vi "AlliGator Decay Fit Parameter Map Context Menu Handler.vi"(8 "Error In":errorcluster, 9 "Decay Fit Parameter":T1, 11 "Image Event Data":T2) -> (0 "Error Out":errorcluster, 3 "AlliGator Actions":T5[](array[typedef]))   [LabVIEW 2021, in "AlliGator Decay Fit Parameter Map.lvlib"]
doc: "Decay Fit Parameter Map contextual menu handler."
uses:
  AlliGator Decay Fit Parameter Map.lvlib
  Action Engine/AlliGator Q Element.ctl
  Action Engine/AlliGator Q Event.ctl
  Image/Image Display Event.ctl
  Image/Image Control Refnum.ctl
  <vilib>/Utility/miscctls.llb/LVPoint32TypeDef.ctl
  Image/Image Display to Clipboard Options.ctl
  Fits/IRF(X)PSED/Decay Fit Parameters & Derived Quantities List v2.ctl
  Globals, Variables, Constants/AlliGator Variables List.ctl
  Files/Load-Save File Info.ctl
  Variant/Variant to Data/Variant to I32.vi
  Action Engine/AlliGator Action Engine.lvlib
  Image/Image.lvlib
  Files/Files.lvlib
  Globals, Variables, Constants/AlliGator Globals, Variables & Constants.lvlib
  Variant/Variant to Data/Variant to Data.lvlib
  Fits/Fits.lvlib
  AlliGator Decay Parameter Map Update Event Data.ctl
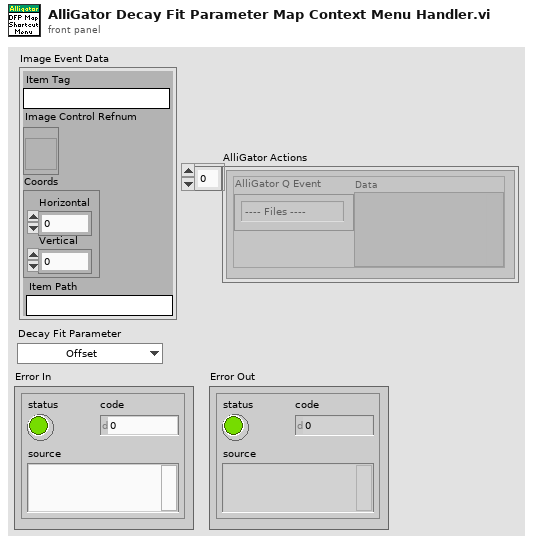
[diagram p1: front panel]
types:
  T1 = typedef "Fits.lvlib/Decay Fit Parameters & Derived Quantities List v2.ctl" = enum16{"Offset", "Baseline", "A_1", "tau_1", "A_2", "tau_2", "<tau>_a", "f1_a", "f2_a", "<tau>_i", "f1_i", "f2_i", "-", "R^2", "Chi^2"}
  T2 = typedef "Image.lvlib/Image Display Event.ctl" = cluster{"Item Tag":string, "Image Control Refnum":T3, "Coords":T4, "Item Path":string}
  T3 = typedef "Image.lvlib/Image Control Refnum.ctl" = refnum<vi>
  T4 = typedef "LVPoint32TypeDef.ctl" = cluster{"Horizontal":i32, "Vertical":i32}
  T5 = typedef "AlliGator Action Engine.lvlib/AlliGator Q Element.ctl" = cluster{"AlliGator Q Event":T6, "Data":variant}
  T6 = typedef "AlliGator Action Engine.lvlib/AlliGator Q Event.ctl" = enum16{"---- Files ----", "Files:Set Batch Export Files To Save", "Files:Set Dataset Loading & Pre-processing Options", "Files:Check #Frames in Dataset", "Files:Increment Frame Index", "Files:Open Mask Image", "Files:Open White Light Image", "Files:Open Single Dataset", "Files:New Folder of Folders Selected", "Files:Load File (all Types)_Scriptable", "Files:Move Flattened Series to Folders Series", "Files:Select Folder", "Files:Load FLI Dataset", "Files:Load Swiss SPAD 1 Dataset", "Files:Load Swiss SPAD 2 Dataset", "Files:Load .sdt FLI Dataset", "Files:Load .ptu FLI Dataset", "Files:Load .bin FLI Dataset", "Files:Load Single Gate Image Folder", "Files:Load I/m/phi Dataset (deprecated)", "Files:Load Single Image", "Files:Subtract Background File", "Files:Export FLI Dataset", "Files:Load HDF5 FLI Dataset", "Files:Set Destination File Path", "Files:Save Mask Image", "Files:Batch Conversion", "Files:New Folder Selected", "Files:Close FLI Dataset", "Files:Close FLI Dataset Series", "Files:Close White Light Image", "Files:Close Mask Image", "---- FLI Dataset ----", "FLI Dataset:Channel Arithmetic", "FLI Dataset:Export Average Lifetime Map as ASCII", "FLI Dataset:Export User-Defined Quantity Map as ASCII", "FLI Dataset:Python Function FLI Dataset Event", "FLI Dataset:ROI Analysis", "FLI Dataset:Tilted Logistic Square Gated IRF Characteristics Map", "FLI Dataset:Logistic Square Gated IRF Characteristics Map", "FLI Dataset:Square Gated IRF Characteristics Map", "FLI Dataset:Multi-ROI Single-Pixel Phasor Analysis", "FLI Dataset:Multi-ROI Single-Pixel NLSF Analysis", "FLI Dataset:All ROIs IRF Extraction", "FLI Dataset:All ROIs Decay Fit Non-Interactive (Fast + Individual IRF)", "FLI Dataset:All ROIs Phasor Analysis", "FLI Dataset:All ROIs Decay Fit", "FLI Dataset:Fluorescence Decay Statistics", "FLI Dataset:Update Decay Statistics Graph", "FLI Dataset:Get Decay from ROI", "FLI Dataset:All ROIs Average Lifetimes", "FLI Dataset:Save/Load Local IRFs", "FLI Dataset:Clear Local IRFs", "---- FLI Dataset Series ----", "FLI Dataset Series:Sum All Datasets in Series", "FLI Dataset Series:Add Dataset to Accumulated Dataset", "FLI Dataset Series:Display Accumulated Dataset", "FLI Dataset Series:Clear Dataset Series Sum", "FLI Dataset Series:Time-Series Analysis (NLSF)", "FLI Dataset Series:Time-Series Analysis (Phasor)", "---- Image ----", "Image:Update Image Profile Plots", "Image:Image Histogram Cursor Move", "Image:Image Histogram", "Image:Image Contrast", "Image:Set Image Histogram Cursor Move Flag", "Image:Clear Image Overlay", "Image:Use ROI as Search Area", "Image:Set ROI Diameter", "Image:Save Image Data as TIFF", "Image:Save Displayed Image with Overlay", "Image:Save Image Overlay Only", "Image:Save Image as Hot Pixel Mask", "Image:Change Source Image Color Palette", "Image:Copy Image to Clipboard", "Image:Source Image ROI Selection", "Image:Delete All ROIs", "Image:Delete All Unselected ROIs", "Image:Delete ROI", "Image:Merge All ROIs", "Image:Store ROI", "Image:Source Image ROI Storage", "Image:Export ROI Description to Notebook", "Image:Save ROI", "Image:Load ROI", "Image:Paste ROI Definition", "Image:Clear ROI", "Image:Identify ROIs in Mask Image", "Image:Create Complementary ROI", "Image:Create Contour ROI", "Image:Create ROI(s) from Pixels with Peak above Min_Scriptable", "Image:Create ROI(s) from Pixels with Intensity above Min_Scriptable", "Image:Compute ROI Statistics", "Image:Delete ROI(s) based on ROI Characteristics", "Image:Create ROI Grid", "Image:ROI to Individual Pixel ROIs", "Image:Python Function Source Image Event", "Image:Show Phasor Calibration Map ROI Centers", "Image:Convert ROI to Mask Image", "Image:Mouse Move", "Image:Mouse Up", "Image:Set Source Image Mouse Move Flag", "Image:Add Scale Bar Overlay", "Image:Delete Existing ROIs Option", "Image:Overlay ROI Median", "Image:Check Current ROI", "---- Decay ----", "Decay:Clear IRF/Reference Plot", "Decay:Add Decay to Graph", "Decay:Smoothen Plot", "Decay:Smoothen Plot Tail", "Decay:Average Selected Plots", "Decay:Extract IRF", "Decay:Optimal IRF Extraction", "Decay:Threshold IRF", "Decay:Fit to Model IRF", "Decay:Fit IRF to Square Gate", "Decay:Fit IRF to Logistic Square Gate", "Decay:Fit IRF to Tilted Logistic Square Gate", "Decay:Create Bounding Cursors Set", "Decay:Export Bounding Cursors Definition to Notebook", "Decay:Denoise Plot", "Decay:Compute Cumulative Function", "Decay:Use as Reference Decay", "Decay:Show Reference Decay/IRF", "Decay:Extrapolate Decay", "Decay:Create Head & Tail Bounding Cursors", "Decay:Store Cursor-defined Head & Tail Fractions", "Decay:Rebin Plot", "Decay:1-Normalize Decay", "Decay:[0-1]-Normalize Plot", "Decay:Straighten Decay", "Decay:Shift Decay", "Decay:Fold Decay", "Decay:Fit Decay", "Decay:Global Fit of Selected Decays", "Decay:Post Global Fit Script", "Decay:Add Global Fit Parameters to Graph", "Decay:Add Decay Parameter(s) to Plot (Graph)", "Decay:Export Decay to Phasor Graph", "Decay:Plot Decay Shifts", "Decay:Compute Average Lifetime", "Decay:Plot Convolution", "Decay:Graph Tip Strip Update", "---- Decay Statistics ----", "Decay Statistics:Tip Strip Update", "---- Intensity Time Trace ----", "Intensity Time Trace:Use File Timestamp", "Intensity Time Trace:Load Intensity Corrections File", "Intensity Time Trace:Clear Intensity Corrections File", "Intensity Time Trace:Tip Strip Update", "---- Phasor Plot ----", "Phasor Plot:Build Phasor Plot", "Phasor Plot:Change Phasor Plot Color Palette", "Phasor Plot:Adjust Phasor Plot Display Range", "Phasor Plot:Highlight Image ROI in Phasor Plot", "Phasor Plot:Save Phasor Plot Image with Overlay", "Phasor Plot:Export Complex Phasor Map", "Phasor Plot:Export Phasor Ratio Map", "Phasor Plot:Export Average Lifetime Map", "Phasor Plot:Compute Phase Lifetime Histogram", "Phasor Plot:Compute Phasor Ratio Histogram", "Phasor Plot:Compute Phase Lifetime vs Intensity Scatter Plot", "Phasor Plot:Weber 2-Component Decomposition", "Phasor Plot:Update Phasor Color Map Vertices", "Phasor Plot:Clear Phasor Overlay", "Phasor Plot:Use Segment Extremities as References", "Phasor Plot:Use UC/Segment Intersections as References", "Phasor Plot:Use UC/Principal Axis Intersections as References", "Phasor Plot:Use UC/Linear Fit Intersections as References", "Phasor Plot:Update Phasor Plot Reference", "Phasor Plot:Show Local Phasor Info in Phasor Plot", "Phasor Plot:Update Phasor Plot State", "Phasor Plot:Phasor Plot ROI Storage", "Phasor Plot:Phasor Plot ROI Selection", "Phasor Plot:Python Function Phasor Plot Event", "Phasor Plot:Overlay Phasor ROI, Ratio or Map in Source Image", "Phasor Plot:Compute Decay of Selected Phasors", "Phasor Plot:Phasor at Image Pixel", "Phasor Plot:Mouse Move", "Phasor Plot:Mouse Up", "Phasor Plot:Display Range Mouse Move", "Phasor Plot:Set Mouse Move Flag", "---- Phasor Graph ----", "Phasor Graph:Calibrated Phasor Map Series", "Phasor Graph:Whole Image Phasor Scatter Plot (deprecated)", "Phasor Graph:Get Phasor Value", "Phasor Graph:Create New Phasor Plot Dialog", "Phasor Graph:Update Last Phasor Value", "Phasor Graph:Update Phasor (m, phi)", "Phasor Graph:Remove Single Phasor from Plot", "Phasor Graph:Add Single Phasor to Plot", "Phasor Graph:Remove Phasor Plot", "Phasor Graph:Remove Selected Phasor Plots", "Phasor Graph:Clear Phasor Data", "Phasor Graph:Clear Phasor Graph", "Phasor Graph:Cursor Move", "Phasor Graph:Draw Cursor Connecting Line", "Phasor Graph:Clear Cursor Connecting Line", "Phasor Graph:Find UC Intersection", "Phasor Graph:Use UC/Cursor-Defined Line Intersections", "Phasor Graph:Use Selected Plots Fitted Line/UC Intersections", "Phasor Graph:Use Selected Plots Principal Axis/UC Intersections", "Phasor Graph:Show Single Phasor", "Phasor Graph:Save Single Phasor Plot", "Phasor Graph:Save All Phasor Plots", "Phasor Graph:Load Phasor Plot(s)", "Phasor Graph:Phasor Multiplication", "Phasor Graph:Compute Average Phasor", "Phasor Graph:Compute Multiple Average Phasors (Selected Plots)", "Phasor Graph:Export Single Phasor Plot Phase Lifetimes", "Phasor Graph:Phase Lifetime Trajectory (deprecated)", "Phasor Graph:Phase Lifetime vs Intensity Scatter Plot (deprecated)", "Phasor Graph:Parameter 2 vs Parameter 1 Scatter Plot", "Phasor Graph:Use Cursor n Location", "Phasor Graph:Set Reference n to Current Phase Lifetime Value", "Phasor Graph:Set Reference n to Lifetime Value", "Phasor Graph:Set Cursor n Location", "Phasor Graph:Save Phasor Graph Image", "Phasor Graph:Update SEPL Plot", "Phasor Graph:Export Single Phasor Plot Data", "Phasor Graph:Export Selected Phasor Plots Data", "Phasor Graph:Python Function Phasor Graph Event", "Phasor Graph:Tip Strip Update", "---- Calibration ----", "Calibration:Set Calibration Type", "Calibration:Load/Save Phasor Calibration", "Calibration:Load/Save Phasor Calibration Series", "Calibration:Load/Save Phasor Calibration Map", "Calibration:Use as Calibration", "Calibration:Compute Optimal Calibration from Phasor References", "Calibration:Clear Phasor Calibration", "Calibration:Single Phasor Calibration Information", "Calibration:Use as Calibration Series", "Calibration:Use as Calibration Map", "Calibration:Clear Calibration Series", "Calibration:Phasor Calibration Series Information", "Calibration:Clear Calibration Map", "Calibration:Phasor Calibration Map Information", "Calibration:Apply Phasor Calibration", "Calibration:Update Single Plot Calibration", "Calibration:Update Multiple Plots Calibration", "Calibration:Clear Single Plot Calibration", "Calibration:Clear All Plots Calibrations", "Calibration:Clear Plot(s) Calibration(s)?", "Calibration:Phasor Calibration Maps (# Gates Series)", "---- Phasor Ratio ----", "Phasor Ratio:Clear Reference n", "Phasor Ratio:Toggle Selected Plot(s)  Lock to Reference 1", "Phasor Ratio:Use as Reference n", "Phasor Ratio:Send Reference n to Notebook", "Phasor Ratio:Toggle Selected Plot(s)  Lock to Reference 2", "Phasor Ratio:Compute Phasor Ratio at Mouse Location", "Phasor Ratio:Compute Phasor Plot's Average Phasor Ratio", "Phasor Ratio:Compute Time-Series Phasor Ratios", "Phasor Ratio:Fit Line to Phasor Ratio Plot", "Phasor Ratio:Save References", "Phasor Ratio:Load References", "Phasor Ratio:Update Phasor Reference 1", "Phasor Ratio:Update Phasor Reference 2", "Phasor Ratio:Move Cursor n to Reference n", "Phasor Ratio:Use as Phasor Reference 1 Lifetime", "Phasor Ratio:Use as Phasor Reference 2 Lifetime", "Phasor Ratio:Export Phasor Ratio Map as ASCII", "Phasor Ratio:Tip Strip Update", "---- Lifetime & Other Parameters Graph ----", "Lifetime:Power Law from Intensity Distribution", "---- Decay Fit Parameter Map ----", "Decay Fit Parameter Map:Export ROI NLSF Data as ASCII", "Decay Fit Parameter Map:Set Decay Fit Parameter Map Selection", "Decay Fit Parameter Map:Build Decay Fit Parameter Map", "Decay Fit Parameter Map:Change Decay Fit Parameter Map Color Palette", "Decay Fit Parameter Map:Export Decay Fit Parameter Map Data as ASCII", "Decay Fit Parameter Map:Export All Decay Fit Parameter Maps Data as ASCII", "Decay Fit Parameter Map:Selected Parameter Scatterplot", "Decay Fit Parameter Map:Parameter 2 vs Parameter 1 Scatterplot", "Decay Fit Parameter Map:Save Decay Fit Parameter Map Image", "Decay Fit Parameter Map:Save-Load IRFs & Fit Data", "Decay Fit Parameter Map:Update Local Decay Plots", "Decay Fit Parameter Map:Python Function Decay Fit Parameters Map Event", "Decay Fit Parameter Map:Overlay Decay Fit Parameter Map in Source Image", "Decay Fit Parameter Map:Selected Parameter vs Intensity Scatterplot", "Decay Fit Parameter Map:Mouse Up", "Decay Fit Parameter Map:Display Range Mouse Move", "Decay Fit Parameter Map:Change Map Resolution", "---- Parameter Map ----", "Parameter Map:Export ROI Parameters Data as ASCII", "Parameter Map:Delete Parameter Map Set", "Parameter Map:Update Parameter List", "Parameter Map:Build Parameter Map", "Parameter Map:Change Parameter Map Color Palette", "Parameter Map:Export Parameter Map Data as ASCII", "Parameter Map:Export All Parameter Maps Data as ASCII", "Parameter Map:Selected Parameter Scatterplot", "Parameter Map:Parameter 2 vs Parameter 1 Scatterplot", "Parameter Map:Selected Parameter vs Intensity Scatterplot", "Parameter Map:Save Parameter Map Image", "Parameter Map:Save-Load IRFs & Parameter Maps (TODO)", "Parameter Map:Set Parameter Map Selection", "Parameter Map:Python Function Parameter Map Event", "Parameter Map:Overlay Parameter Map in Source Image", "Parameter Map:Update Local Decay Plots", "Parameter Map:Mouse Up", "Parameter Map:Display Range Mouse Move", "---- Generic Graph ----", "Generic Graph:Generic XY Graph Event", "Generic Graph:Python Function XY Graph Event", "Generic Graph:New Plot", "Generic Graph:Save Plot", "Generic Graph:XY Plot Histogram", "Generic Graph:Set XY Graph Plot Name", "Generic Graph:Set Last Cursor Style", "Generic Graph:Tip Strip Update", "---- GUI ----", "GUI:Start Script", "GUI:Type of Displayed Image Changed", "GUI:Gate Image Slide Changed", "GUI:Show Busy Icon", "GUI:Show Busy Icon & Abort Button", "GUI:Hide Busy Icon", "GUI:Hide Busy Icon & Abort Button", "GUI:Abort", "GUI:End Script", "GUI:Start Timing", "GUI:End Timing", "GUI:Set State Indicator", "GUI:Send Parameters JSON Strings to Clipboard", "GUI:Set Gate Step", "GUI:Idle", "GUI:Initialization", "GUI:Quit", "GUI:Increment Dataset Index", "GUI:Set Dataset Index to -1", "GUI:Time Series Slider Moved", "GUI:Time Series Slider Changed", "GUI:Toggle Playback or Loop", "GUI:Playback Script", "GUI:Set Phasor Frequency", "GUI:Open Window", "GUI:Start Test Script", "GUI:End Test Script", "DEBUG"}
  T7 = typedef "Image.lvlib/Image Display to Clipboard Options.ctl" = cluster{"Include Overlay (T)":bool, "Image Only (T)":bool}
  T8 = cluster{"Fit Parameter 1":T1, "Fit Parameter 2":T1}
  T9 = typedef "AlliGator Globals, Variables & Constants.lvlib/AlliGator Variables List.ctl" = enum16{"---- GUI ----", "GUI:Initialization Status", "GUI:State Indicators Refnum", "GUI:Original AlliGator Menu Items", "GUI:Current Action Loop State", "GUI:Script in progress", "GUI:Playback", "GUI:Loop Playback", "GUI:Search ROI Used", "GUI:Search ROI", "Decay Graph Max Legend Size", "Intensity Graph Max Legend Size", "Decay Statistics Graph Max Legend Size", "Phasor Graph Max Legend Size", "Phasor Ratio Graph Max Legend Size", "Lifetime Graph Max Legend Size", "---- Files ----", "Files:Export Dataset Frames as Individual Files", "Files:Show Batch Export Help Balloons", "Files:Frames in Dataset", "Files:ptu File Frame Start Indices", "Files:Current Frame in Dataset", "Files:Current Frame Timestamp", "Files:Dataset Loaded", "Files:Dataset Metadata", "Files:Dataset Channel", "Files:Dataset Data Description", "Files:Background Dataset Metadata", "Files:Background Dataset Channel", "Files:Background Dataset Data Description", "Files:Background File Subtraction", "Files:Background File Path", "Files:Background File Pile-up Correction", "Files:Background File Pixel Well Capacity", "Files:Background File Scaling Factor", "Files:Current Dataset Load Settings", "Files:Dataset Path", "Files:ICCD-specific Information", "Files:Macrotime Gate Separation", "------ Python Plugins ------", "Python Plugins:Information", "Python Plugins:Python Session", "Python Plugins:Valid Python Session?", "---- Source Image ----", "Source Image:ROIs", "Source Image:Current ROI", "Source Image:ROI Event Refnum", "X_Source Image:Display Range", "X_Source Image:Palette Information", "X_Source Image:Type of Displayed Image", "X_Time Gate Slider", "Source Image:Palette List", "Source Image:Scale", "Source Image:ROI Overlay Color", "Source Image:Overlay to Erase", "Source Image:Is Displayed Image Accumulated", "Source Image:White Light Image Modified", "Source Image:Mask Image Modified", "---- Image Profile Window ----", "Image Profile:Window Event Refnum", "Image Profile:IntensityType", "Image Profile:Intensity Average Type", "Image Profile:Intensity-weighted SDV", "Image Profile:Box Profile Type", "Image Profile:Window Open", "Image Profile:Plotted Fit Parameter", "------ Phasor Graph -------", "Phasor Graph:Show Line", "---- Phasor Plot ---", "Phasor Plot:Parameters Changed", "Phasor Plot:FLI Dataset Modified since last Calculation", "Phasor Harmonics Data", "Selected Phasor Harmonics", "Phasor Harmonic Manager Event Refnum", "Phasor Plot:ROIs", "Phasor Plot:Current ROI", "Phasor Plot:ROI Event Refnum", "Phasor Plot:Image Reference Points", "Phasor Plot:Computed", "Phasor Plot:Palette Information", "Phasor Plot:Palette List", "Phasor Plot:Phasor Ratio Palette Information", "Phasor Plot:Phasor Ratio Palette List", "Phasor Plot:Image Scale", "Phasor Plot:Image Overlay to Erase", "Phasor Plot:Image Elements to Update", "Phasor Plot:Current Calculation Parameters", "Phasor Plot:Current Calibration Options", "Phasor Plot:Reset Cumulated Phasor Plot", "Phasor Plot:Reference 1", "Phasor Plot:Lifetime Reference 1", "Phasor Plot:Reference 1 Frequency", "Phasor Plot:Reference 2", "Phasor Plot:Lifetime Reference 2", "Phasor Plot:Reference 2 Frequency", "---- Decay Analysis ----", "Number of Selected Decays to Fit", "LS Fit Results", "LAR Fit Results", "BS Fit Results", "Last Decay Max - Min", "Best Fit Parameters", "Best Fit Parameter Names", "Actual Size X", "Actual Size Y", "Binning X", "Binning Y", "Actual # Gates", "Dataset Number", "Gates to...", "Gates Skipped", "Gates to keep", "Gate Step", "Gate Separation", "Reversed Gates", "Pile-up Correction", "Pixel Well Capacity", "Background Subtracted", "Background Subtraction Method", "Background Definition Range", "Background File (deprecated)", "Number of Dataset Accumulated", "Array of Accumulated Dataset Paths", "Do Averaged Datasets", "Destination File Path", "Process Plot Target", "Use 1/D as Phasor Frequency", "---- Decay Fit Parameter Map -----", "Decay Fit Parameter Map:Palette Information", "Decay Fit Parameter Map:Palette List", "Decay Fit Parameter Map:X Resolution", "Decay Fit Parameter Map:Y Resolution", "---- Parameter Map ----", "Parameter Map:Palette Information", "Parameter Map:Palette List", "------- Local Decay Window ---------", "Local Decay Graph Window:Event Refnum", "Local Decay Graph Window:Use normalized IRF for convolution", "----- Miscellaneous ----", "Misc:Skippable Dialog Windows Status"}
  T10 = typedef "Files.lvlib/Load-Save File Info.ctl" = cluster{"Load/Save":bool, "File Path":path}
  T11 = typedef "AlliGator Decay Fit Parameter Map.lvlib/AlliGator Decay Parameter Map Update Event Data.ctl" = cluster{"Parameter":T1, "Parameter changed":bool}
  T12 = cluster{"Image Control Refnum":T3, "Image to Clipboard Options":T7}
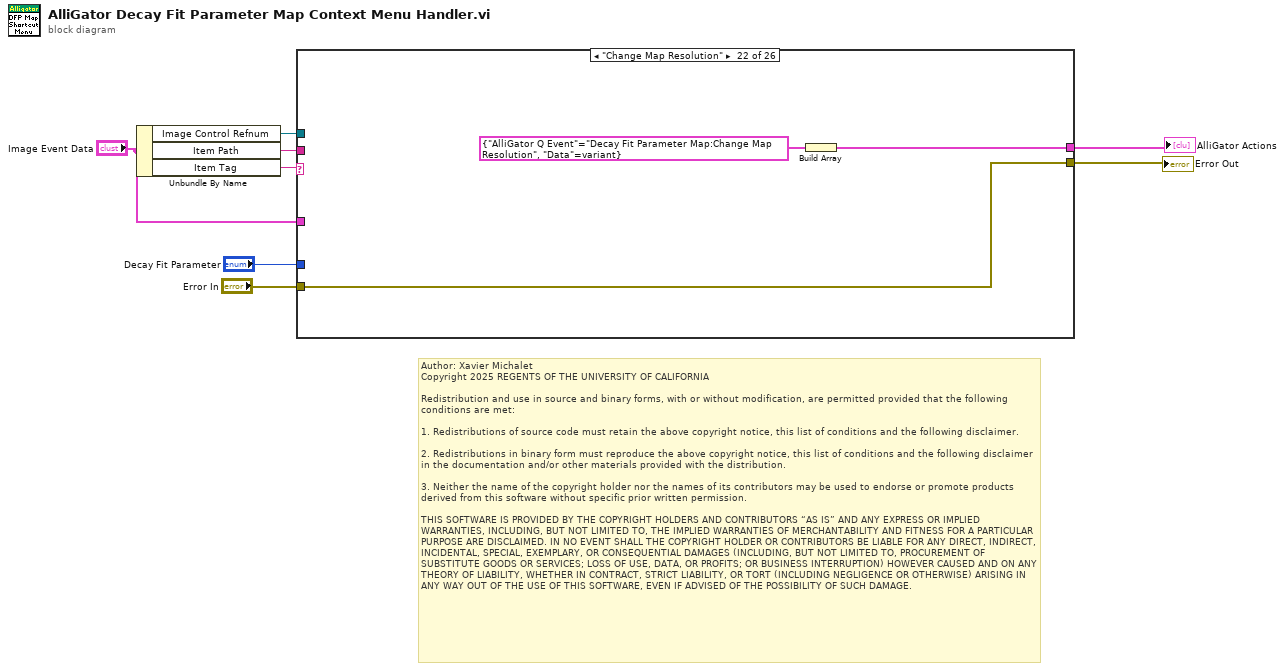
[diagram p0: block diagram]
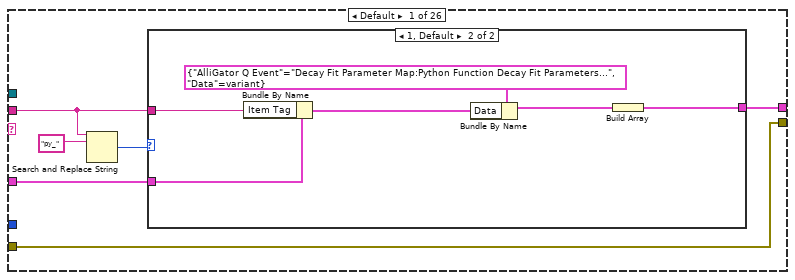
[diagram p2: hidden frame]
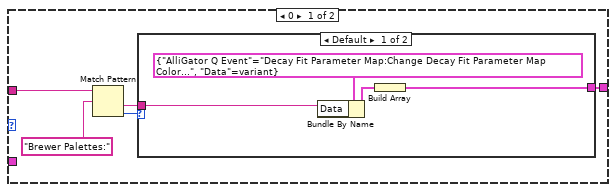
[diagram p3: hidden frame]
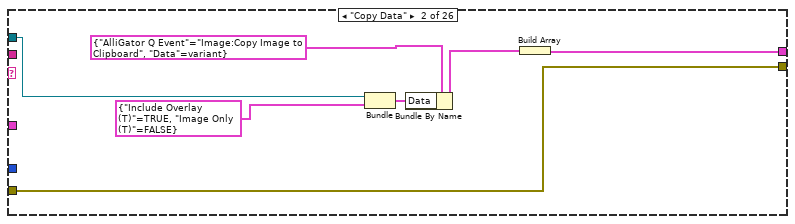
[diagram p5: hidden frame]
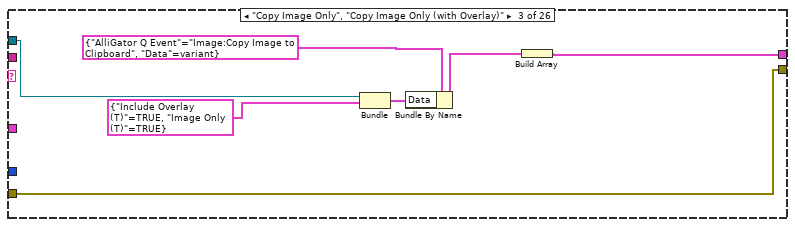
[diagram p6: hidden frame]
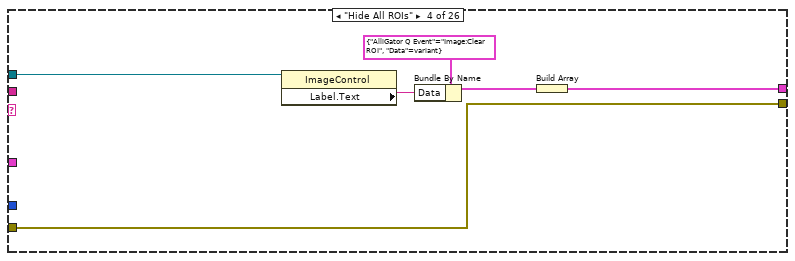
[diagram p7: hidden frame]
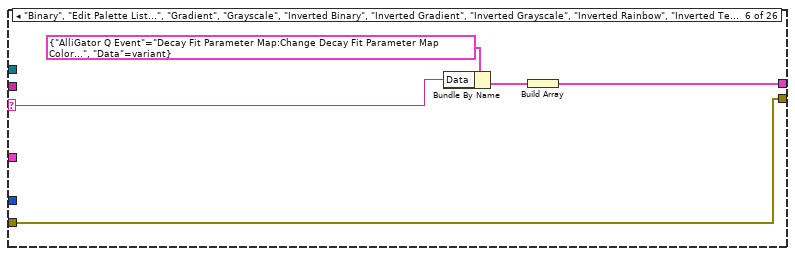
[diagram p9: hidden frame]
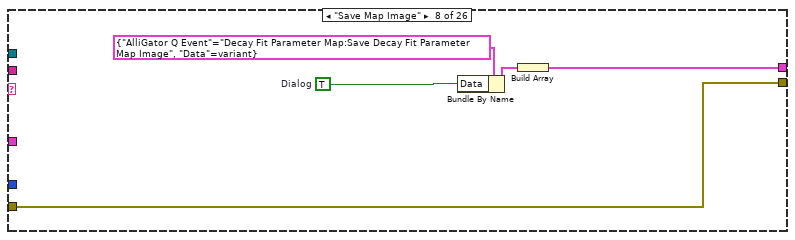
[diagram p11: hidden frame]
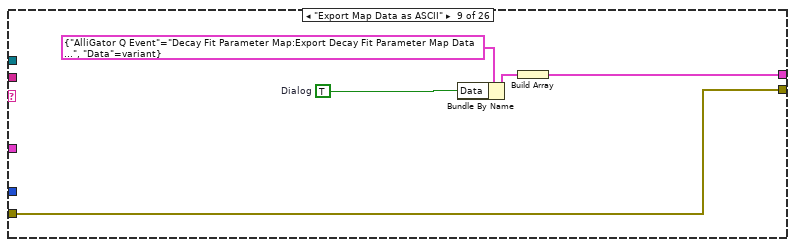
[diagram p12: hidden frame]
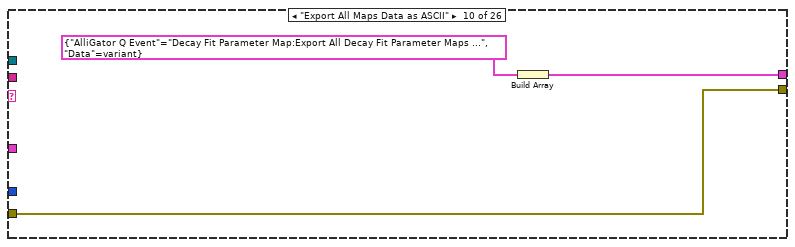
[diagram p13: hidden frame]
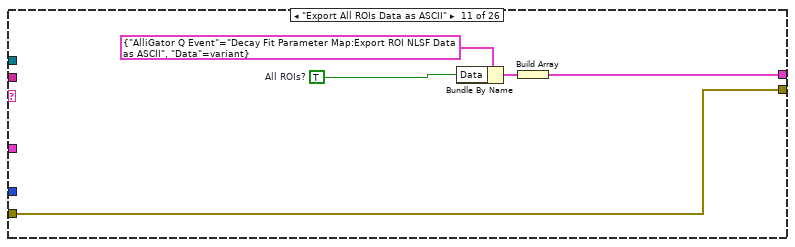
[diagram p14: hidden frame]
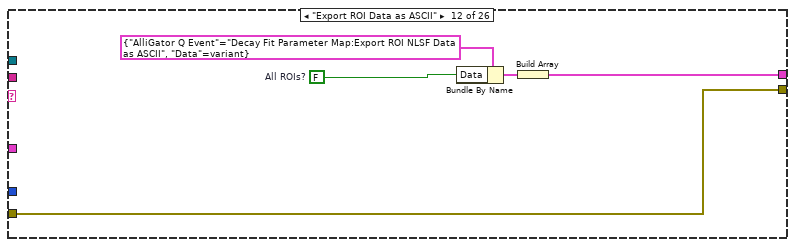
[diagram p15: hidden frame]
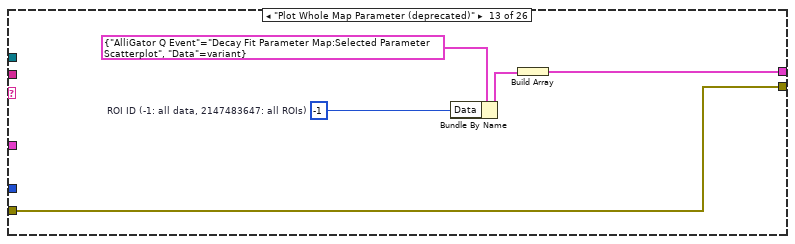
[diagram p16: hidden frame]
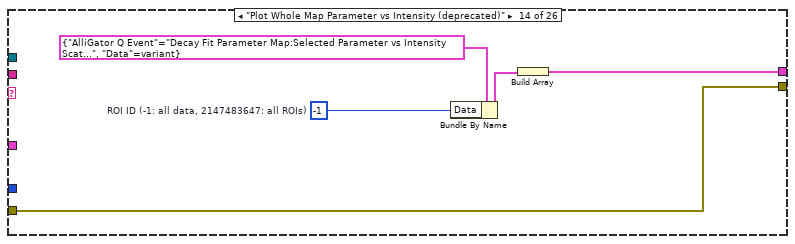
[diagram p17: hidden frame]
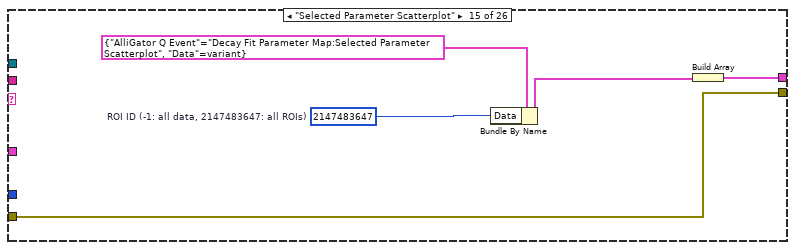
[diagram p18: hidden frame]
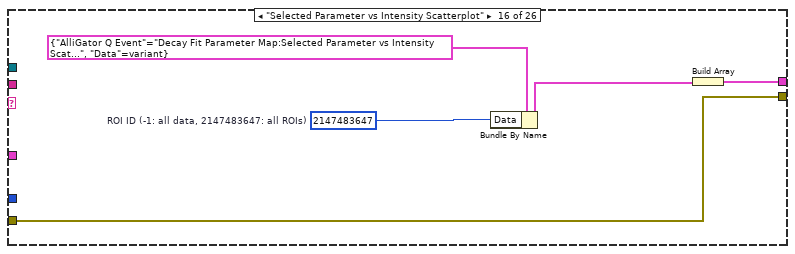
[diagram p19: hidden frame]
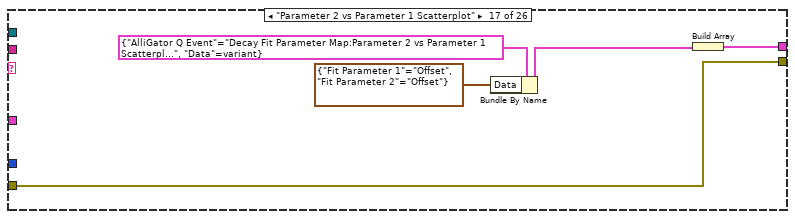
[diagram p20: hidden frame]
diagram:
  # "Author: Xavier Michalet\nCopyright 2025 REGENTS OF THE UNIVERSITY OF CALIFORNIA\n\nRedistribution and use in source and binary forms, with or without modification, are permitted provided that the following conditions are met:\n\n1. Redistributions of source code must retain the above copyright notice, this list of conditions and the following disclaimer.\n\n2. Redistributions in binary form must reproduce the above copyright notice, this list of conditions and the following disclaimer in the documentation and/or other materials provided with the distribution.\n\n3. Neither the name of the copyright holder nor the names of its contributors may be used to endorse or promote products derived from this software without specific prior written permission.\n\nTHIS SOFTWARE IS PROVIDED BY THE COPYRIGHT HOLDERS AND CONTRIBUTORS “AS IS” AND ANY EXPRESS OR IMPLIED WARRANTIES, INCLUDING, BUT NOT LIMITED TO, THE IMPLIED WARRANTIES OF MERCHANTABILITY AND FITNESS FOR A PARTICULAR PURPOSE ARE DISCLAIMED. IN NO EVENT SHALL THE COPYRIGHT HOLDER OR CONTRIBUTORS BE LIABLE FOR ANY DIRECT, INDIRECT, INCIDENTAL, SPECIAL, EXEMPLARY, OR CONSEQUENTIAL DAMAGES (INCLUDING, BUT NOT LIMITED TO, PROCUREMENT OF SUBSTITUTE GOODS OR SERVICES; LOSS OF USE, DATA, OR PROFITS; OR BUSINESS INTERRUPTION) HOWEVER CAUSED AND ON ANY THEORY OF LIABILITY, WHETHER IN CONTRACT, STRICT LIABILITY, OR TORT (INCLUDING NEGLIGENCE OR OTHERWISE) ARISING IN ANY WAY OUT OF THE USE OF THIS SOFTWARE, EVEN IF ADVISED OF THE POSSIBILITY OF SUCH DAMAGE."
  n1 = Unbundle By Name("Image Event Data") -> ("Image Control Refnum"=w5:T3, "Item Path"=w4:string, "Item Tag"=w3:string)
  n2 = case shown="\"Change Map Resolution\"" w3 {
    selector: w3 -> [_ _ _ _ _ w53 _ _ _ _ _ _ _ _ _ _ _ _ _ _ _ _ _ _ _ _]
    tunnel: w5 -> [_ w32 w39 w44 _ _ _ _ _ _ _ _ _ _ _ _ _ _ _ _ _ _ _ _ w151 w153]
    tunnel: w4 -> [w9 _ _ _ _ _ _ _ _ _ _ _ _ _ _ _ _ _ _ _ _ _ _ _ _ _]
    tunnel: [w14 w31 w38 w45 _ w52 _ w58 w63 w68 w73 w78 w83 w88 w93 w98 w103 w112 w120 w127 w135 w138 w141 _ _ _] -> w8
    tunnel: "Error In" -> [w13 w30 w37 w49 w50 w51 w56 w61 w66 w69 w74 w79 w84 w89 w94 w99 w104 w108 w116 w128 w136 w139 w147 w148 w149 w152]
    tunnel: [w13 w30 w37 w49 w50 w51 w56 w61 w66 w69 w74 w79 w84 w89 w94 w99 w104 w107 w115 w128 w136 w139 w147 w148 w149 w152] -> w6
    tunnel: "Image Event Data" -> [w10 _ _ _ _ _ _ _ _ _ _ _ _ _ _ _ _ _ _ _ _ _ _ _ _ _]
    tunnel: "Decay Fit Parameter" -> [_ _ _ _ _ _ _ _ _ _ _ _ _ _ _ _ _ _ _ _ _ _ w140 _ _ _]
    frame Default {
      n3 = Search and Replace String(input string=w9, search string="py_") -> (number of replacements=w11:i32)  [unwired: 6 in, 3 out]
      n4 = case shown="1, Default" w11 {
        tunnel: [w16 w24] -> w14
        tunnel: w9 -> [w15 w27]
        tunnel: w10 -> [_ w25]
        frame 0 {
          n5 = Match Pattern(string=w15, regular expression="Brewer Palettes:") -> (after substring=w17:string, offset past match=w18:i32)  [unwired: 1 in, 2 out]
          n6 = case shown="Default" w18 {
            tunnel: w17 -> [w21 _]
            tunnel: [w20 _] -> w16
            frame Default {
              n7 = Bundle By Name(cluster=T5 {"AlliGator Q Event"=enum."Decay Fit Parameter Map:Change Decay Fit Parameter Map Color Palette", "Data"=variant} ("element"), "Data"=w21) -> (w22:T5)
              n8 = Build Array(w22) -> (w20:T5[])
            }
            frame -1 {
            }
          }
        }
        frame 1, Default {
          n9 = Bundle By Name(cluster=w25, "Item Tag"=w27) -> (w28:T2)
          n10 = Bundle By Name(cluster=T5 {"AlliGator Q Event"=enum."Decay Fit Parameter Map:Python Function Decay Fit Parameters Map Event", "Data"=variant}, "Data"=w28) -> (w26:T5)
          n11 = Build Array(w26) -> (w24:T5[])
        }
      }
    }
    frame "Copy Data" {
      n12 = Bundle("Image Control Refnum"=w32, "Image to Clipboard Options"=T7 {"Include Overlay (T)"=TRUE, "Image Only (T)"=FALSE}) -> (w33:T12)  [unwired: 1 in]
      n13 = Bundle By Name(cluster=T5 {"AlliGator Q Event"=enum."Image:Copy Image to Clipboard", "Data"=variant} ("element"), "Data"=w33) -> (w35:T5)
      n14 = Build Array(w35) -> (w31:T5[])
    }
    frame "Copy Image Only", "Copy Image Only (with Overlay)" {
      n15 = Bundle("Image Control Refnum"=w39, "Image to Clipboard Options"=T7 {"Include Overlay (T)"=TRUE, "Image Only (T)"=TRUE}) -> (w40:T12)  [unwired: 1 in]
      n16 = Bundle By Name(cluster=T5 {"AlliGator Q Event"=enum."Image:Copy Image to Clipboard", "Data"=variant} ("element"), "Data"=w40) -> (w42:T5)
      n17 = Build Array(w42) -> (w38:T5[])
    }
    frame "Hide All ROIs" {
      n18 = property class="ImageControl"(reference=w44) -> ("Label.Text"=w46:string)  [unwired: 1 in, 2 out]
      n19 = Bundle By Name(cluster=T5 {"AlliGator Q Event"=enum."Image:Clear ROI", "Data"=variant} ("element"), "Data"=w46) -> (w47:T5)
      n20 = Build Array(w47) -> (w45:T5[])
    }
    frame "---------Palette----------" {
    }
    frame "Binary", "Edit Palette List...", "Gradient", "Grayscale", "Inverted Binary", "Inverted Gradient", "Inverted Grayscale", "Inverted Rainbow", "Inverted Temperature", "Rainbow", "Select New Palette...", "Temperature" {
      n21 = Bundle By Name(cluster=T5 {"AlliGator Q Event"=enum."Decay Fit Parameter Map:Change Decay Fit Parameter Map Color Palette", "Data"=variant} ("element"), "Data"=w53) -> (w54:T5)
      n22 = Build Array(w54) -> (w52:T5[])
    }
    frame "--------- Others  ---------" {
    }
    frame "Save Map Image" {
      w57 = TRUE  # Dialog
      n23 = Bundle By Name(cluster=T5 {"AlliGator Q Event"=enum."Decay Fit Parameter Map:Save Decay Fit Parameter Map Image", "Data"=variant} ("Time-Gated Phasor Q Element"), "Data"=w57) -> (w59:T5)
      n24 = Build Array(w59) -> (w58:T5[])
    }
    frame "Export Map Data as ASCII" {
      w62 = TRUE  # Dialog
      n25 = Bundle By Name(cluster=T5 {"AlliGator Q Event"=enum."Decay Fit Parameter Map:Export Decay Fit Parameter Map Data as ASCII", "Data"=variant} ("Time-Gated Phasor Q Element"), "Data"=w62) -> (w64:T5)
      n26 = Build Array(w64) -> (w63:T5[])
    }
    frame "Export All Maps Data as ASCII" {
      n27 = Build Array(T5 {"AlliGator Q Event"=enum."Decay Fit Parameter Map:Export All Decay Fit Parameter Maps Data as ASCII", "Data"=variant} ("Time-Gated Phasor Q Element")) -> (w68:T5[])
    }
    frame "Export All ROIs Data as ASCII" {
      w70 = TRUE  # All ROIs?
      n28 = Bundle By Name(cluster=T5 {"AlliGator Q Event"=enum."Decay Fit Parameter Map:Export ROI NLSF Data as ASCII", "Data"=variant} ("Time-Gated Phasor Q Element"), "Data"=w70) -> (w71:T5)
      n29 = Build Array(w71) -> (w73:T5[])
    }
    frame "Export ROI Data as ASCII" {
      w75 = FALSE  # All ROIs?
      n30 = Bundle By Name(cluster=T5 {"AlliGator Q Event"=enum."Decay Fit Parameter Map:Export ROI NLSF Data as ASCII", "Data"=variant} ("Time-Gated Phasor Q Element"), "Data"=w75) -> (w76:T5)
      n31 = Build Array(w76) -> (w78:T5[])
    }
    frame "Plot Whole Map Parameter (deprecated)" {
      w80 = -1  # ROI ID (-1: all data, 2147483647: all ROIs)
      n32 = Bundle By Name(cluster=T5 {"AlliGator Q Event"=enum."Decay Fit Parameter Map:Selected Parameter Scatterplot", "Data"=variant} ("Time-Gated Phasor Q Element"), "Data"=w80) -> (w81:T5)
      n33 = Build Array(w81) -> (w83:T5[])
    }
    frame "Plot Whole Map Parameter vs Intensity (deprecated)" {
      w85 = -1  # ROI ID (-1: all data, 2147483647: all ROIs)
      n34 = Bundle By Name(cluster=T5 {"AlliGator Q Event"=enum."Decay Fit Parameter Map:Selected Parameter vs Intensity Scatterplot", "Data"=variant} ("Time-Gated Phasor Q Element"), "Data"=w85) -> (w86:T5)
      n35 = Build Array(w86) -> (w88:T5[])
    }
    frame "Selected Parameter Scatterplot" {
      w90 = 2147483647  # ROI ID (-1: all data, 2147483647: all ROIs)
      n36 = Bundle By Name(cluster=T5 {"AlliGator Q Event"=enum."Decay Fit Parameter Map:Selected Parameter Scatterplot", "Data"=variant} ("Time-Gated Phasor Q Element"), "Data"=w90) -> (w91:T5)
      n37 = Build Array(w91) -> (w93:T5[])
    }
    frame "Selected Parameter vs Intensity Scatterplot" {
      w95 = 2147483647  # ROI ID (-1: all data, 2147483647: all ROIs)
      n38 = Bundle By Name(cluster=T5 {"AlliGator Q Event"=enum."Decay Fit Parameter Map:Selected Parameter vs Intensity Scatterplot", "Data"=variant} ("Time-Gated Phasor Q Element"), "Data"=w95) -> (w96:T5)
      n39 = Build Array(w96) -> (w98:T5[])
    }
    frame "Parameter 2 vs Parameter 1 Scatterplot" {
      n40 = Bundle By Name(cluster=T5 {"AlliGator Q Event"=enum."Decay Fit Parameter Map:Parameter 2 vs Parameter 1 Scatterplot", "Data"=variant} ("Time-Gated Phasor Q Element"), "Data"=T8 {"Fit Parameter 1"=enum."Offset", "Fit Parameter 2"=enum."Offset"}) -> (w101:T5)
      n41 = Build Array(w101) -> (w103:T5[])
    }
    frame "Plot Selected ROI(s) Parameter (deprecated)" {
      n42 = call "Alligator Variables Storage.vi"("AlliGator Variable"=AlliGator_Variables_List."Source Image:Current ROI" ("Alligator Variable"), "Error In"=w108) -> ("Error Out"=w107:errorcluster, "Data out"=w109:variant)  [unwired: 7 in, 1 out]
      n43 = call-poly "Variant to Data.vi"("Variant"=w109) -> ("Value"=w105:i32)  [unwired: 8 in]
      n44 = Bundle By Name(cluster=T5 {"AlliGator Q Event"=enum."Decay Fit Parameter Map:Selected Parameter Scatterplot", "Data"=variant} ("Time-Gated Phasor Q Element"), "Data"=w105) -> (w110:T5)
      n45 = Build Array(w110) -> (w112:T5[])
    }
    frame "Plot Selected ROI(s) Parameter vs Intensity (deprecated)" {
      n46 = call "Alligator Variables Storage.vi"("AlliGator Variable"=AlliGator_Variables_List."Source Image:Current ROI" ("Alligator Variable"), "Error In"=w116) -> ("Error Out"=w115:errorcluster, "Data out"=w117:variant)  [unwired: 7 in, 1 out]
      n47 = call-poly "Variant to Data.vi"("Variant"=w117) -> ("Value"=w113:i32)  [unwired: 8 in]
      n48 = Bundle By Name(cluster=T5 {"AlliGator Q Event"=enum."Decay Fit Parameter Map:Selected Parameter vs Intensity Scatterplot", "Data"=variant} ("Time-Gated Phasor Q Element"), "Data"=w113) -> (w118:T5)
      n49 = Build Array(w118) -> (w120:T5[])
    }
    frame "Save IRFs & Fit Data" {
      n50 = Bundle By Name(cluster=T10 {"Load/Save"=FALSE, "File Path"=path ""} ("Calibration File Information"), "File Path"=path "", "Load/Save"=TRUE) -> (w122:T10)
      n51 = Bundle By Name(cluster=T5 {"AlliGator Q Event"=enum."Decay Fit Parameter Map:Save-Load IRFs & Fit Data", "Data"=variant} ("Time-Gated Phasor Q Element"), "Data"=w122) -> (w125:T5)
      n52 = Build Array(w125) -> (w127:T5[])
    }
    frame "Load IRFs & Fit Data" {
      n53 = Bundle By Name(cluster=T10 {"Load/Save"=FALSE, "File Path"=path ""} ("Calibration File Information"), "File Path"=path "", "Load/Save"=FALSE) -> (w132:T10)
      n54 = Bundle By Name(cluster=T5 {"AlliGator Q Event"=enum."Decay Fit Parameter Map:Save-Load IRFs & Fit Data", "Data"=variant} ("Time-Gated Phasor Q Element"), "Data"=w132) -> (w133:T5)
      n55 = Build Array(w133) -> (w135:T5[])
    }
    frame "Change Map Resolution" {
      n56 = Build Array(T5 {"AlliGator Q Event"=enum."Decay Fit Parameter Map:Change Map Resolution", "Data"=variant} ("Time-Gated Phasor Q Element")) -> (w138:T5[])
    }
    frame "Refresh Image" {
      w143 = TRUE  # Parameter changed
      n57 = Bundle(cluster=T11 {"Parameter"=enum."Offset", "Parameter changed"=FALSE} ("output cluster"), "Parameter"=w140, "Parameter changed"=w143) -> (w142:T11)
      n58 = Bundle By Name(cluster=T5 {"AlliGator Q Event"=enum."Decay Fit Parameter Map:Build Decay Fit Parameter Map", "Data"=variant} ("Time-Gated Phasor Q Element"), "Data"=w142) -> (w145:T5)
      n59 = Build Array(w145) -> (w141:T5[])
    }
    frame "--------------" {
    }
    frame "Zoom to Fit" {
      n60 = call "Image Display Zoom to Fit.vi"("Keep Aspect Ratio (T)"=FALSE, "Display Image Control Refnum"=w151) -> ()  [unwired: 9 in, 1 out]
    }
    frame "Zoom to Fit (Keep Aspect Ratio)" {
      n61 = call "Image Display Zoom to Fit.vi"("Display Image Control Refnum"=w153) -> ()  [unwired: 10 in, 1 out]
    }
  }
  "Error Out" <- w6
  "AlliGator Actions" <- w8
